vi "TagMetadataToImage.vi"(8 "error in (no error)":errorcluster, 10 "Image In":T1, 11 "Device in":refnum<class "Device.lvclass">) -> (0 "error out":errorcluster, 2 "Image Out":T1, 3 "Device out":refnum<class "Device.lvclass">)   [LabVIEW 2020]
uses:
  Device.lvclass
  <vilib>/vision/Image Controls.llb/IMAQ Image.ctl
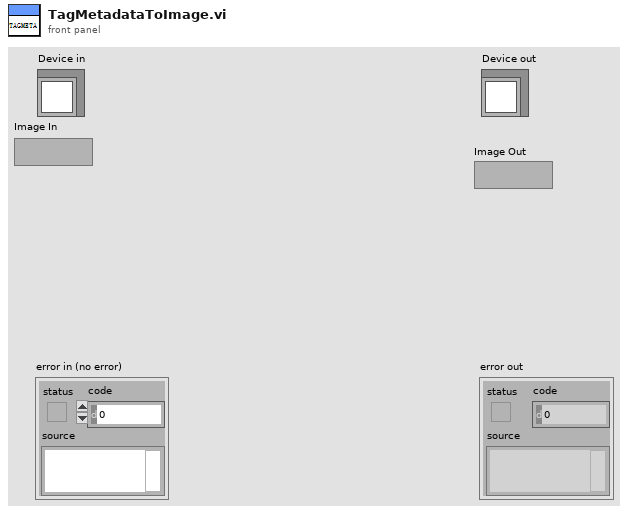
[diagram p1: front panel]
types:
  T1 = typedef "IMAQ Image.ctl" = refnum<image>
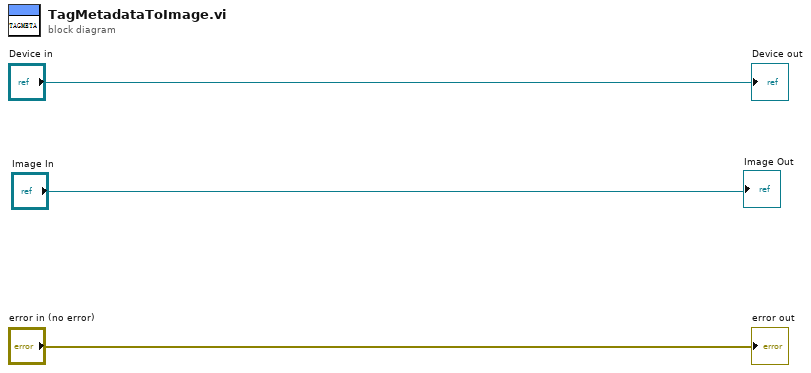
[diagram p0: block diagram]
diagram:
  "error out" <- "error in (no error)"
  "Device out" <- "Device in"
  "Image Out" <- "Image In"
